vi "Digital Control Loop.vi"(8 "error in (no error)":errorcluster, 11 "Message Queues":T1) -> (0 "error out":errorcluster)   [LabVIEW 2014, in "PLS Digital Control.lvlib"]
doc: "Message loop for handling messages pertaining to the acquisition of data from the hardware."
uses:
  PLS Digital Control.lvlib
  support/Message Queue/All Message Queues.ctl
  support/Message Queue/Message Cluster.ctl
  Hardware Configuration.ctl
  Acquisition State.ctl
  Internal event.ctl
  <vilib>/Utility/error.llb/whitespace.ctl
  start info.ctl
  type de test.ctl
  <vilib>/DAQmx/write.llb/DAQmx Write (Digital 1D Bool NChan 1Samp 1Line).vi
  <vilib>/DAQmx/read.llb/DAQmx Read (Digital 1D Bool NChan 1Samp 1Line).vi
  GLB_Timing.vi
  support/Message Queue/Enqueue Message (Single).vi
  support/Message Queue/Enqueue Message (Array).vi
  <vilib>/DAQmx/miscellaneous.llb/DAQmx Fill In Error Info.vi
  <vilib>/Utility/error.llb/Error Cluster From Error Code.vi
  <vilib>/ErrorRing/Error Ring.xnode
  support/Message Queue/PLS Message Queue.lvlib
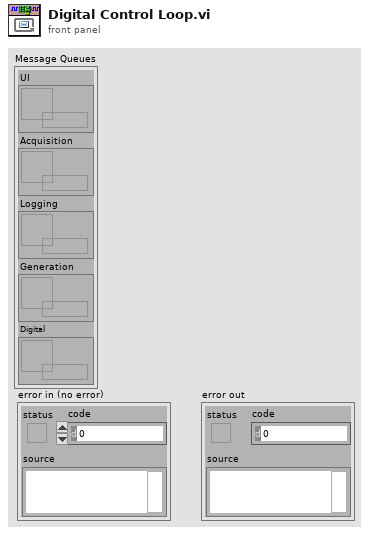
[diagram p1: front panel]
types:
  T1 = typedef "PLS Message Queue.lvlib/All Message Queues.ctl" = cluster{"UI":refnum<queue>, "Acquisition":refnum<queue>, "Logging":refnum<queue>, "Generation":refnum<queue>, "Digital":refnum<queue>}
  T2 = typedef "PLS Digital Control.lvlib/Hardware Configuration.ctl" = cluster{"DO":cluster{"task name":string, "task_ref":refnum<k21>, "lines":tag}}
  T3 = typedef "PLS Digital Control.lvlib/Acquisition State.ctl" = enum16{"Idle", "Ready"}
  T4 = typedef "start info.ctl" = cluster{"type":T5, "ligne index":i32}
  T5 = typedef "type de test.ctl" = enum16{"Eau froide - standard", "Eau chaude", "Chocs thermiques"}
  T6 = cluster{"actif?":bool, "t0":timestamp, "timing":cluster{"Tcold":dbl, "Twarm":dbl}, "froid?":bool}
  T7 = cluster{"actif?":bool, "t0":timestamp, "timing":cluster{"Topen":dbl, "Tclose":dbl}, "belier":bool}
  T8 = typedef "PLS Digital Control.lvlib/Internal event.ctl" = cluster{"cmd":string, "Ligne":i32}
  T9 = typedef "whitespace.ctl" = u16
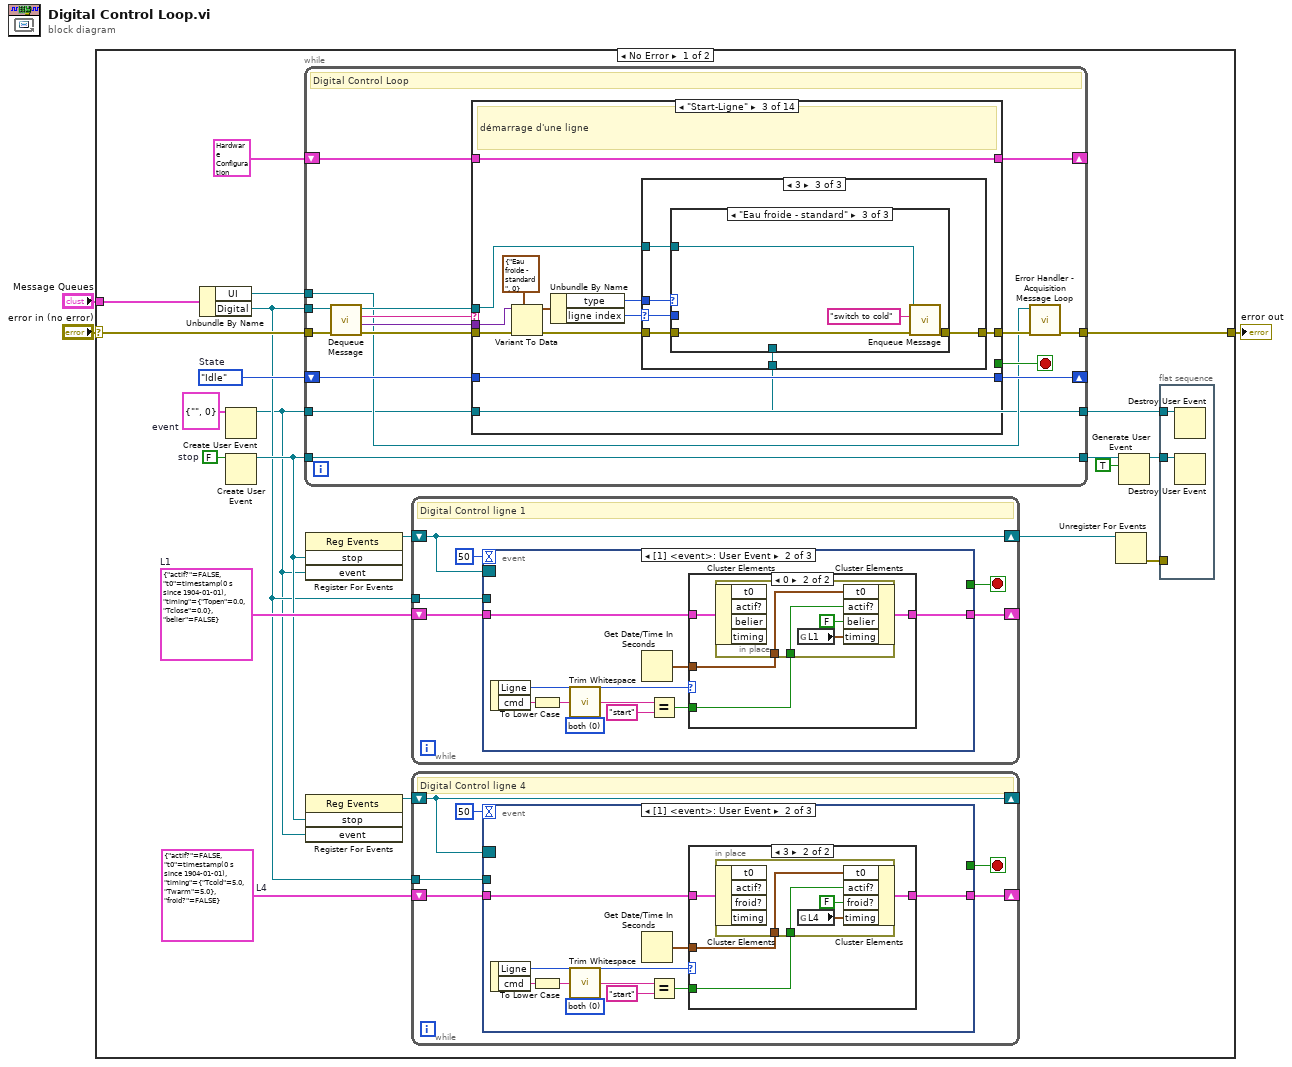
[diagram p0: block diagram]
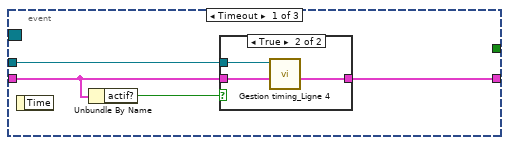
[diagram p2: hidden frame]
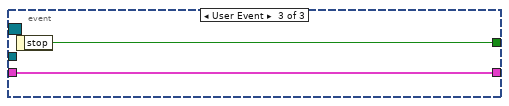
[diagram p5: hidden frame]
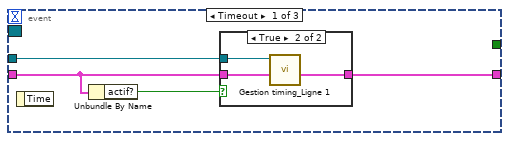
[diagram p6: hidden frame]
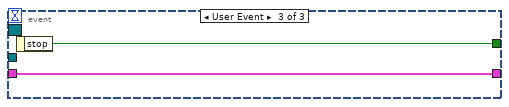
[diagram p9: hidden frame]
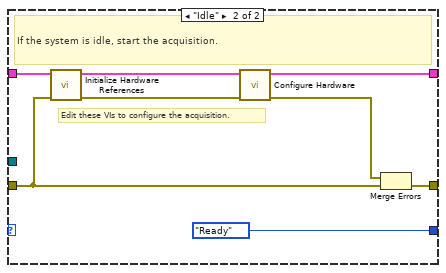
[diagram p12: hidden frame]
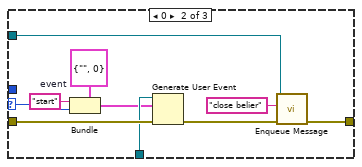
[diagram p14: hidden frame]
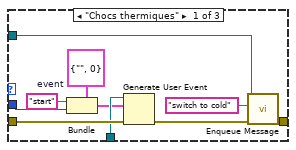
[diagram p15: hidden frame]
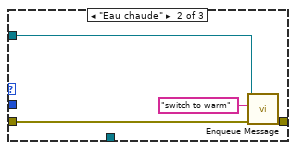
[diagram p16: hidden frame]
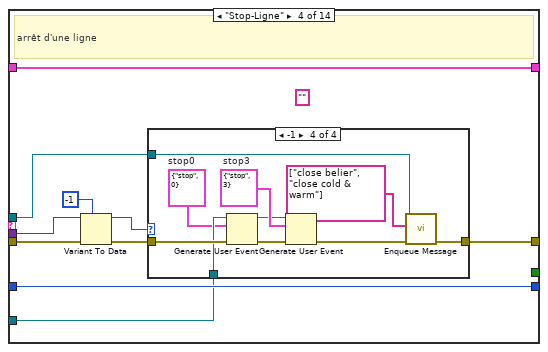
[diagram p17: hidden frame]
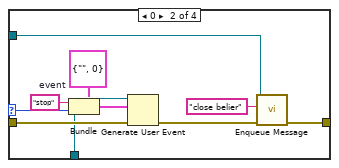
[diagram p19: hidden frame]
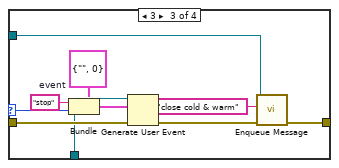
[diagram p20: hidden frame]
diagram:
  n1 = case shown="No Error" "error in (no error)" {
    selector: "error in (no error)" -> [w21 w323]
    tunnel: "Message Queues" -> [w24 _]
    tunnel: [w23 w323] -> w2
    frame No Error {
      w5 = T6 {"actif?"=FALSE, "t0"=timestamp(0 s since 1904-01-01), "timing"={"Tcold"=5.0, "Twarm"=5.0}, "froid?"=FALSE}  # L4
      w9 = T7 {"actif?"=FALSE, "t0"=timestamp(0 s since 1904-01-01), "timing"={"Topen"=0.0, "Tclose"=0.0}, "belier"=FALSE}  # L1
      w11 = T8 {"cmd"="", "Ligne"=0}  # event
      w18 = FALSE  # stop
      w20 = Acquisition_State."Idle"  # State
      n2 = Unbundle By Name(w24) -> ("UI"=w19:refnum<queue>, "Digital"=w6:refnum<queue>)
      n3 = Create User Event(user event datatype=w11) -> (user event=w4:refnum<user-event>)  [unwired: 1 in, 1 out]
      n4 = Create User Event(user event datatype=w18) -> (user event=w7:refnum<user-event>)  [unwired: 1 in, 1 out]
      n5 = while {
        tunnel: w6 -> [w105]
        shift-right: [w111] -> _
        shift-left: T2 {"DO"={"task name"="DO", "task_ref"="", "lines"="Dev1/port0/line2:3, Dev1/port0/line5"}} ("Data Cluster") -> [w112]
        tunnel: w19 -> [w99]
        shift-right: [w103] -> _
        shift-left: w20 -> [w104]
        tunnel: w21 -> [w109]
        tunnel: [w102] -> w23
        tunnel: w7 -> [w98]
        tunnel: [w98] -> w14
        tunnel: w4 -> [w97]
        tunnel: [w97] -> w10
        stop <- w110 stop-if-true
        # "Digital Control Loop"
        n6 = call "Dequeue Message.vi"("error in (no error)"=w109, "Message Queue"=w105) -> ("error out"=w108:errorcluster, "Message Data"=w106:variant, "Message"=w107:string, "dup Message Queue"=w100:refnum<queue>)  [unwired: 6 in]
        n7 = case "Message Cases" shown="\"Start-Ligne\"" w107 {
          selector: w107 -> [_ _ _ _ _ _ _ _ _ _ _ _ _ w312]
          tunnel: w100 -> [_ w119 w137 w181 _ _ w243 _ _ _ _ _ _ _]
          tunnel: w108 -> [w115 w120 w143 w187 w226 w237 w245 _ _ _ _ _ _ _]
          tunnel: [w115 w122 w138 w188 w227 w241 w247 w250 w265 _ w284 w296 _ w313] -> w101
          tunnel: w112 -> [w114 w121 w145 w190 w224 w235 w246 w256 w266 w275 w285 w297 w308 w315]
          tunnel: [w114 w118 w145 w190 w224 w234 w246 w256 w266 w275 w285 w297 w308 w315] -> w111
          tunnel: [_ _ _ _ _ _ TRUE _ _ _ _ _ _ _] -> w110
          tunnel: w106 -> [_ _ w141 w185 _ w240 _ w255 _ _ _ _ _ _]
          tunnel: w104 -> [w113 w116 w144 w189 w223 w236 w242 w257 w267 w276 w286 w298 w309 w314]
          tunnel: [w113 w117 w144 w189 w222 w236 w242 w257 w267 w276 w286 w298 w309 w314] -> w103
          tunnel: w97 -> [_ _ w140 w183 _ _ _ _ _ _ _ _ _ _]
          frame "Initialize" {
            # "Initialize  - Initialize is currently a no-op.  The hardware initialization takes place in the 'Start' message."
          }
          frame "Start" {
            # "Start - Configure and start the acquisition."
            n8 = case shown="\"Ready\"" w116 {
              selector: w116 -> [w123 _]
              tunnel: [w124 w133] -> w122
              tunnel: w121 -> [w125 w132]
              tunnel: w120 -> [w124 w126]
              tunnel: w119 -> [_ _]
              tunnel: [w125 w128] -> w118
              tunnel: [w123 Acquisition_State."Ready" ("Acquisition State")] -> w117
              frame "Ready" {
                # "The system is already acquiring. Ignore the \"Start\" message."
              }
              frame "Idle" {
                # "Edit these VIs to configure the acquisition."
                # "If the system is idle, start the acquisition."
                n9 = call "Initialize Hardware References.vi"("error in (no error)"=w126, "Hardware Resources in"=w132) -> ("error out"=w131:errorcluster, "Hardware Resources out"=w129:T2)  [unwired: 8 in]
                n10 = call "Configure Hardware.vi"("error in (no error)"=w131, "Hardware Resources in"=w129) -> ("error out"=w130:errorcluster, "Hardware Resources out"=w128:T2)  [unwired: 8 in]
                n11 = Merge Errors(w130, w126) -> (w133:errorcluster)
              }
            }
          }
          frame "Start-Ligne" {
            # "démarrage d'une ligne"
            n12 = Variant To Data(error in=w143, type=T4 {"type"=enum."Eau froide - standard", "ligne index"=0} ("start info"), Variant=w141) -> (data=w139:T4, error out=w142:errorcluster)
            n13 = Unbundle By Name(w139) -> ("type"=w134:T5, "ligne index"=w135:i32)
            n14 = case shown="3" w135 {
              selector: w135 -> [_ w151 w160]
              tunnel: [w146 w147 w158] -> w138
              tunnel: w142 -> [w146 w156 w162]
              tunnel: w140 -> [_ w155 w161]
              tunnel: w137 -> [_ w149 w159]
              tunnel: w134 -> [_ _ w157]
              frame Default {
              }
              frame 0 {
                w153 = T8 {"cmd"="", "Ligne"=0}  # event
                n15 = Bundle(cluster=w153, "cmd"="start", "Ligne"=w151) -> (w154:T8)
                n16 = Generate User Event(user event=w155, event data cluster=w154, error in=w156) -> (error out=w148:errorcluster)  [unwired: 1 in, 1 out]
                n17 = call-poly "Enqueue Message.vi"("error in (no error)"=w148, "Message"="close belier", "Message Queue"=w149) -> ("error out"=w147:errorcluster)  [unwired: 7 in, 1 out]
              }
              frame 3 {
                n18 = case shown="\"Eau froide - standard\"" w157 {
                  tunnel: w162 -> [w172 w173 w177]
                  tunnel: w161 -> [w171 _ _]
                  tunnel: w160 -> [w167 _ _]
                  tunnel: w159 -> [w165 w175 w179]
                  tunnel: [w163 w174 w178] -> w158
                  frame "Chocs thermiques" {
                    w169 = T8 {"cmd"="", "Ligne"=0}  # event
                    n19 = Bundle(cluster=w169, "cmd"="start", "Ligne"=w167) -> (w170:T8)
                    n20 = Generate User Event(user event=w171, event data cluster=w170, error in=w172) -> (error out=w164:errorcluster)  [unwired: 1 in, 1 out]
                    n21 = call-poly "Enqueue Message.vi"("error in (no error)"=w164, "Message"="switch to cold", "Message Queue"=w165) -> ("error out"=w163:errorcluster)  [unwired: 7 in, 1 out]
                  }
                  frame "Eau chaude" {
                    n22 = call-poly "Enqueue Message.vi"("error in (no error)"=w173, "Message"="switch to warm", "Message Queue"=w175) -> ("error out"=w174:errorcluster)  [unwired: 7 in, 1 out]
                  }
                  frame "Eau froide - standard" {
                    n23 = call-poly "Enqueue Message.vi"("error in (no error)"=w177, "Message"="switch to cold", "Message Queue"=w179) -> ("error out"=w178:errorcluster)  [unwired: 7 in, 1 out]
                  }
                }
              }
            }
          }
          frame "Stop-Ligne" {
            (unwired) "" ("Message")
            # "arrêt d'une ligne"
            n24 = Variant To Data(error in=w187, type=-1, Variant=w185) -> (data=w182:i32, error out=w186:errorcluster)
            n25 = case shown="-1" w182 {
              selector: w182 -> [_ w196 w206 _]
              tunnel: [w191 w193 w203 w214] -> w188
              tunnel: w186 -> [w191 w201 w211 w221]
              tunnel: w183 -> [_ w200 w210 w220]
              tunnel: w181 -> [_ w192 w202 w213]
              frame Default {
              }
              frame 0 {
                w198 = T8 {"cmd"="", "Ligne"=0}  # event
                n26 = Bundle(cluster=w198, "cmd"="stop", "Ligne"=w196) -> (w199:T8)
                n27 = Generate User Event(user event=w200, event data cluster=w199, error in=w201) -> (error out=w194:errorcluster)  [unwired: 1 in, 1 out]
                n28 = call-poly "Enqueue Message.vi"("error in (no error)"=w194, "Message"="close belier", "Message Queue"=w192) -> ("error out"=w193:errorcluster)  [unwired: 7 in, 1 out]
              }
              frame 3 {
                w208 = T8 {"cmd"="", "Ligne"=0}  # event
                n29 = Bundle(cluster=w208, "cmd"="stop", "Ligne"=w206) -> (w209:T8)
                n30 = Generate User Event(user event=w210, event data cluster=w209, error in=w211) -> (error out=w204:errorcluster)  [unwired: 1 in, 1 out]
                n31 = call-poly "Enqueue Message.vi"("error in (no error)"=w204, "Message"="close cold & warm", "Message Queue"=w202) -> ("error out"=w203:errorcluster)  [unwired: 7 in, 1 out]
              }
              frame -1 {
                w217 = T8 {"cmd"="stop", "Ligne"=3}  # stop3
                w218 = T8 {"cmd"="stop", "Ligne"=0}  # stop0
                n32 = Generate User Event(user event=w220, event data cluster=w218, error in=w221) -> (user event out=w216:refnum<user-event>, error out=w219:errorcluster)  [unwired: 1 in]
                n33 = Generate User Event(user event=w216, event data cluster=w217, error in=w219) -> (error out=w215:errorcluster)  [unwired: 1 in, 1 out]
                n34 = call-poly "Enqueue Message.vi"("error in (no error)"=w215, "Message Array"=string[] ["close belier", "close cold & warm"], "Message Queue"=w213) -> ("error out"=w214:errorcluster)  [unwired: 7 in, 1 out]
              }
            }
          }
          frame "Stop" {
            # "Stop - Stop the Acquisition."
            n35 = case shown="\"Ready\"" w223 {
              selector: w223 -> [w228 _]
              tunnel: w226 -> [w229 w233]
              tunnel: [w229 w230] -> w225
              tunnel: w224 -> [_ w232]
              tunnel: [w228 Acquisition_State."Idle" ("State")] -> w222
              frame "Idle" {
                # "The system is already idle. Ignore the \"Stop\" message."
              }
              frame "Ready" {
                # "If the system is acquiring, stop the acquisition."
                n36 = call "Stop Acquisition.vi"("error in (no error)"=w233, "Hardware Resources in"=w232) -> ("error out"=w230:errorcluster)  [unwired: 9 in]
              }
            }
            n37 = Merge Errors(w225) -> (w227:errorcluster)
          }
          frame "Update Settings" {
            # "New settings are available, update the current ones stored in the shift register with the settings sent as part of the message"
            n38 = Variant To Data(error in=w237, type=w235, Variant=w240) -> (data=w238:T2, error out=w239:errorcluster)
            n39 = Select(t=w235, s=w239, f=w238) -> (s? t:f=w234:T2)
            n40 = Merge Errors(w237) -> (w241:errorcluster)
          }
          frame "Exit" {
            # "Release the Acquisition queue reference"
            # "Stop the VI"
            # "Exit - Send the Exit message to the UI Message Handler."
            n41 = Release Queue(queue=w243, error in (no error)=w245) -> (error out=w244:errorcluster)  [unwired: 1 in, 2 out]
            n42 = Merge Errors(w244) -> (w247:errorcluster)
          }
          frame "port" {
            # "change on port"
            n43 = Variant To Data(type=bool[] [], Variant=w255) -> (data=w253:bool[], error out=w251:errorcluster)  [unwired: 1 in]
            n44 = Unbundle By Name(w256) -> ("DO.task_ref"=w252:refnum<k21>)
            n45 = call-poly <vilib>:"DAQmx Write.vi"("task/channels in"=w252, "data"=w253, "timeout"=0.1, "error in"=w251) -> ("error out"=w250:errorcluster)  [unwired: 9 in, 2 out]
          }
          frame "open belier" {
            # "ouverture de la vanne bélier"
            n46 = Unbundle By Name(w266) -> ("DO.task_ref"=w263:refnum<k21>)
            n47 = call-poly <vilib>:"DAQmx Read.vi"("task/channels in"=w263) -> ("task out"=w262:refnum<k21>, "data"=w261:bool[])  [unwired: 12 in, 1 out]
            n48 = Replace Array Subset(array=w261, new element=TRUE ("new element/subarray"), index=2) -> (w260:bool[])
            n49 = call-poly <vilib>:"DAQmx Write.vi"("task/channels in"=w262, "data"=w260, "timeout"=0.1) -> ("error out"=w265:errorcluster)  [unwired: 10 in, 2 out]
          }
          frame "close belier" {
            # "fermeture de la vanne bélier"
            n50 = Unbundle By Name(w275) -> ("DO.task_ref"=w273:refnum<k21>)
            n51 = call-poly <vilib>:"DAQmx Read.vi"("task/channels in"=w273) -> ("task out"=w272:refnum<k21>, "data"=w271:bool[])  [unwired: 12 in, 1 out]
            n52 = Replace Array Subset(array=w271, new element=FALSE ("new element/subarray"), index=2) -> (w270:bool[])
            n53 = call-poly <vilib>:"DAQmx Write.vi"("task/channels in"=w272, "data"=w270, "timeout"=0.1) -> ()  [unwired: 10 in, 3 out]
          }
          frame "switch to cold" {
            # "passage à l'eau froide sur ligne 4"
            n54 = Unbundle By Name(w285) -> ("DO.task_ref"=w282:refnum<k21>)
            n55 = call-poly <vilib>:"DAQmx Read.vi"("task/channels in"=w282) -> ("task out"=w281:refnum<k21>, "data"=w280:bool[])  [unwired: 12 in, 1 out]
            n56 = in-place {
              n57 = in-place-array #1(w280, 0, 1) -> ()  [unwired: 2 out]
              n58 = in-place-array #1(FALSE ("element"), TRUE ("element")) -> (w279:bool[])  [unwired: 2 out]
            }
            n59 = call-poly <vilib>:"DAQmx Write.vi"("task/channels in"=w281, "data"=w279, "timeout"=0.1) -> ("error out"=w284:errorcluster)  [unwired: 10 in, 2 out]
          }
          frame "switch to warm" {
            # "passage à l'eau chaude sur ligne 4"
            n60 = Unbundle By Name(w297) -> ("DO.task_ref"=w294:refnum<k21>)
            n61 = call-poly <vilib>:"DAQmx Read.vi"("task/channels in"=w294) -> ("task out"=w293:refnum<k21>, "data"=w292:bool[])  [unwired: 12 in, 1 out]
            n62 = in-place {
              n63 = in-place-array #2(w292, 0, 1) -> ()  [unwired: 2 out]
              n64 = in-place-array #2(TRUE ("element"), FALSE ("element")) -> (w291:bool[])  [unwired: 2 out]
            }
            n65 = call-poly <vilib>:"DAQmx Write.vi"("task/channels in"=w293, "data"=w291, "timeout"=0.1) -> ("error out"=w296:errorcluster)  [unwired: 10 in, 2 out]
          }
          frame "close cold & warm" {
            # "fermeture des 2 vannes"
            n66 = Unbundle By Name(w308) -> ("DO.task_ref"=w306:refnum<k21>)
            n67 = call-poly <vilib>:"DAQmx Read.vi"("task/channels in"=w306) -> ("task out"=w305:refnum<k21>, "data"=w304:bool[])  [unwired: 12 in, 1 out]
            n68 = in-place {
              n69 = in-place-array #3(w304, 0, 1) -> ()  [unwired: 2 out]
              n70 = in-place-array #3(FALSE ("element"), FALSE ("element")) -> (w303:bool[])  [unwired: 2 out]
            }
            n71 = call-poly <vilib>:"DAQmx Write.vi"("task/channels in"=w305, "data"=w303, "timeout"=0.1) -> ()  [unwired: 10 in, 3 out]
          }
          frame Default {
            # "'Default' case only runs if there is a message that isn't defined in any of the other cases.  Output a programming error."
            n72 = xnode "Error Ring"("parameter 0"=w312) -> ("error out"=w313:errorcluster)
          }
        }
        n73 = call "Error Handler - Acquisition Message Loop.vi"("error in (no error)"=w101, "Message Queue"=w99) -> ("dup error in"=w102:errorcluster)  [unwired: 8 in, 1 out]
      }
      n74 = register-events(w7, w4) -> (reference out=w17:refnum<event-registration>)  [unwired: 2 in, 1 out]
      n75 = register-events(w7, w4) -> (reference out=w8:refnum<event-registration>)  [unwired: 2 in, 1 out]
      n76 = while {
        shift-right: [w66] -> w16
        shift-left: w17 -> [w66]
        shift-right: [w64] -> _
        shift-left: w9 -> [w63]
        tunnel: w6 -> [w62]
        stop <- w65 stop-if-true
        # "Digital Control ligne 1"
        n77 = event shown="[1] <event>: User Event" {
          selector: w66 -> [_ _ _]
          dyn-events: _ -> [_ _ _]
          timeout: 50 -> [_ _ _]
          tunnel: [_ _ w96] -> w65
          tunnel: [w68 w84 w95] -> w64
          tunnel: w63 -> [w69 w85 w95]
          tunnel: w62 -> [w70 _ _]
          event Timeout {
            n78 = event-data() -> ()  [unwired: 1 in, 1 out]
            n79 = Unbundle By Name(w69) -> ("actif?"=w71:bool)
            n80 = case shown="True" w71 {
              tunnel: w70 -> [_ w75]
              tunnel: w69 -> [w72 w74]
              tunnel: [w72 w73] -> w68
              frame False {
              }
              frame True {
                n81 = call "Gestion timing_Ligne 1.vi"("L1 in"=w74, "Queue in"=w75) -> ("L1 out"=w73:T7)  [unwired: 9 in]
              }
            }
          }
          event User Event {
            w80 = T9 0 items=["both", "start of string", "end of string"] ("location (both)")
            n82 = event-data() -> ("Ligne"=w77:i32, "cmd"=w83:string)  [unwired: 1 in]
            n83 = To Lower Case(string=w83) -> (all lower case string=w82:string)
            n84 = call <vilib>:"Trim Whitespace.vi"("string"=w82, "location (both)"=w80) -> ("trimmed string"=w81:string)
            n85 = Get Date/Time In Seconds() -> (seconds since 1Jan1904=w76:timestamp)
            n86 = Equal?(x=w81, y="start" ("x")) -> (x = y?=w78:bool)
            n87 = case shown="0" w77 {
              tunnel: w85 -> [w86 w90]
              tunnel: [w86 w89] -> w84
              tunnel: w78 -> [_ w88]
              tunnel: w76 -> [_ w87]
              frame Default {
              }
              frame 0 {
                n88 = in-place {
                  in-place-border: w88 -> [w93]
                  in-place-border: w87 -> [w94]
                  n89 = in-place-cluster #4(w90) -> ()  [unwired: 4 out]
                  n90 = global read "GLB_Timing.vi" "L1"() -> (w92:cluster{"Topen":dbl, "Tclose":dbl})
                  n91 = in-place-cluster #4("t0"=w94, "actif?"=w93, "belier"=FALSE, "timing"=w92) -> (w89:T7)
                }
              }
            }
          }
          event User Event {
            n92 = event-data() -> ("stop"=w96:bool)  [unwired: 1 in]
          }
        }
      }
      n93 = while {
        shift-right: [w29] -> _
        shift-left: w8 -> [w29]
        shift-right: [w27] -> _
        shift-left: w5 -> [w26]
        tunnel: w6 -> [w25]
        stop <- w28 stop-if-true
        # "Digital Control ligne 4"
        n94 = event shown="[1] <event>: User Event" {
          selector: w29 -> [_ _ _]
          dyn-events: _ -> [_ _ _]
          timeout: 50 -> [_ _ _]
          tunnel: [_ _ w59] -> w28
          tunnel: [w31 w47 w58] -> w27
          tunnel: w26 -> [w32 w48 w58]
          tunnel: w25 -> [w33 _ _]
          event Timeout {
            n95 = event-data() -> ()  [unwired: 1 in, 1 out]
            n96 = Unbundle By Name(w32) -> ("actif?"=w34:bool)
            n97 = case shown="True" w34 {
              tunnel: w33 -> [_ w38]
              tunnel: w32 -> [w35 w36]
              tunnel: [w35 w37] -> w31
              frame False {
              }
              frame True {
                n98 = call "Gestion timing_Ligne 4.vi"("L4 in"=w36, "Queue in"=w38) -> ("L4 out"=w37:T6)  [unwired: 9 in]
              }
            }
          }
          event User Event {
            w43 = T9 0 items=["both", "start of string", "end of string"] ("location (both)")
            n99 = event-data() -> ("Ligne"=w40:i32, "cmd"=w46:string)  [unwired: 1 in]
            n100 = To Lower Case(string=w46) -> (all lower case string=w45:string)
            n101 = call <vilib>:"Trim Whitespace.vi"("string"=w45, "location (both)"=w43) -> ("trimmed string"=w44:string)
            n102 = Get Date/Time In Seconds() -> (seconds since 1Jan1904=w39:timestamp)
            n103 = Equal?(x=w44, y="start" ("x")) -> (x = y?=w41:bool)
            n104 = case shown="3" w40 {
              tunnel: w48 -> [w49 w53]
              tunnel: [w49 w52] -> w47
              tunnel: w41 -> [_ w51]
              tunnel: w39 -> [_ w50]
              frame Default {
              }
              frame 3 {
                n105 = in-place {
                  in-place-border: w51 -> [w56]
                  in-place-border: w50 -> [w57]
                  n106 = in-place-cluster #5(w53) -> ()  [unwired: 4 out]
                  n107 = global read "GLB_Timing.vi" "L4"() -> (w54:cluster{"Tcold":dbl, "Twarm":dbl})
                  n108 = in-place-cluster #5("t0"=w57, "actif?"=w56, "froid?"=FALSE ("belier"), "timing"=w54) -> (w52:T6)
                }
              }
            }
          }
          event User Event {
            n109 = event-data() -> ("stop"=w59:bool)  [unwired: 1 in]
          }
        }
      }
      n110 = Unregister For Events(event registration refnum=w16) -> (error out=w15:errorcluster)  [unwired: 1 in]
      n111 = Generate User Event(user event=w14, event data cluster=TRUE ("event data")) -> (user event out=w13:refnum<user-event>)  [unwired: 2 in, 1 out]
      n112 = flat-sequence {
        tunnel: w15 -> [_]
        tunnel: w13 -> [w61]
        tunnel: w10 -> [w60]
        frame #0 {
          n113 = Destroy User Event(user event=w60) -> ()  [unwired: 1 in, 1 out]
          n114 = Destroy User Event(user event=w61) -> ()  [unwired: 1 in, 1 out]
        }
      }
    }
    frame Error {
    }
  }
  "error out" <- w2
